vi "Spindle_load_RT_truncated_one(SubVI).vi"() -> (3 "Z_position":string)   [LabVIEW 2017]
uses:
  <vilib>/regexp/Match Regular Expression.xnode
  <vilib>/addons/internet/NI_InternetTK_Core_VIs.lvlib
panel:
  out "speed 3":string
  out "speed 2":string
  out "speed":string
  in  "String 2":string="http://amrcmtconnect.shef.ac.uk:5000/DMU40EVO/current"
  out "content 7":string
  out "after match":string
  out "error out":errorcluster
  out "content 4":string
  out "X_position":string
  out "Y_poistion":string
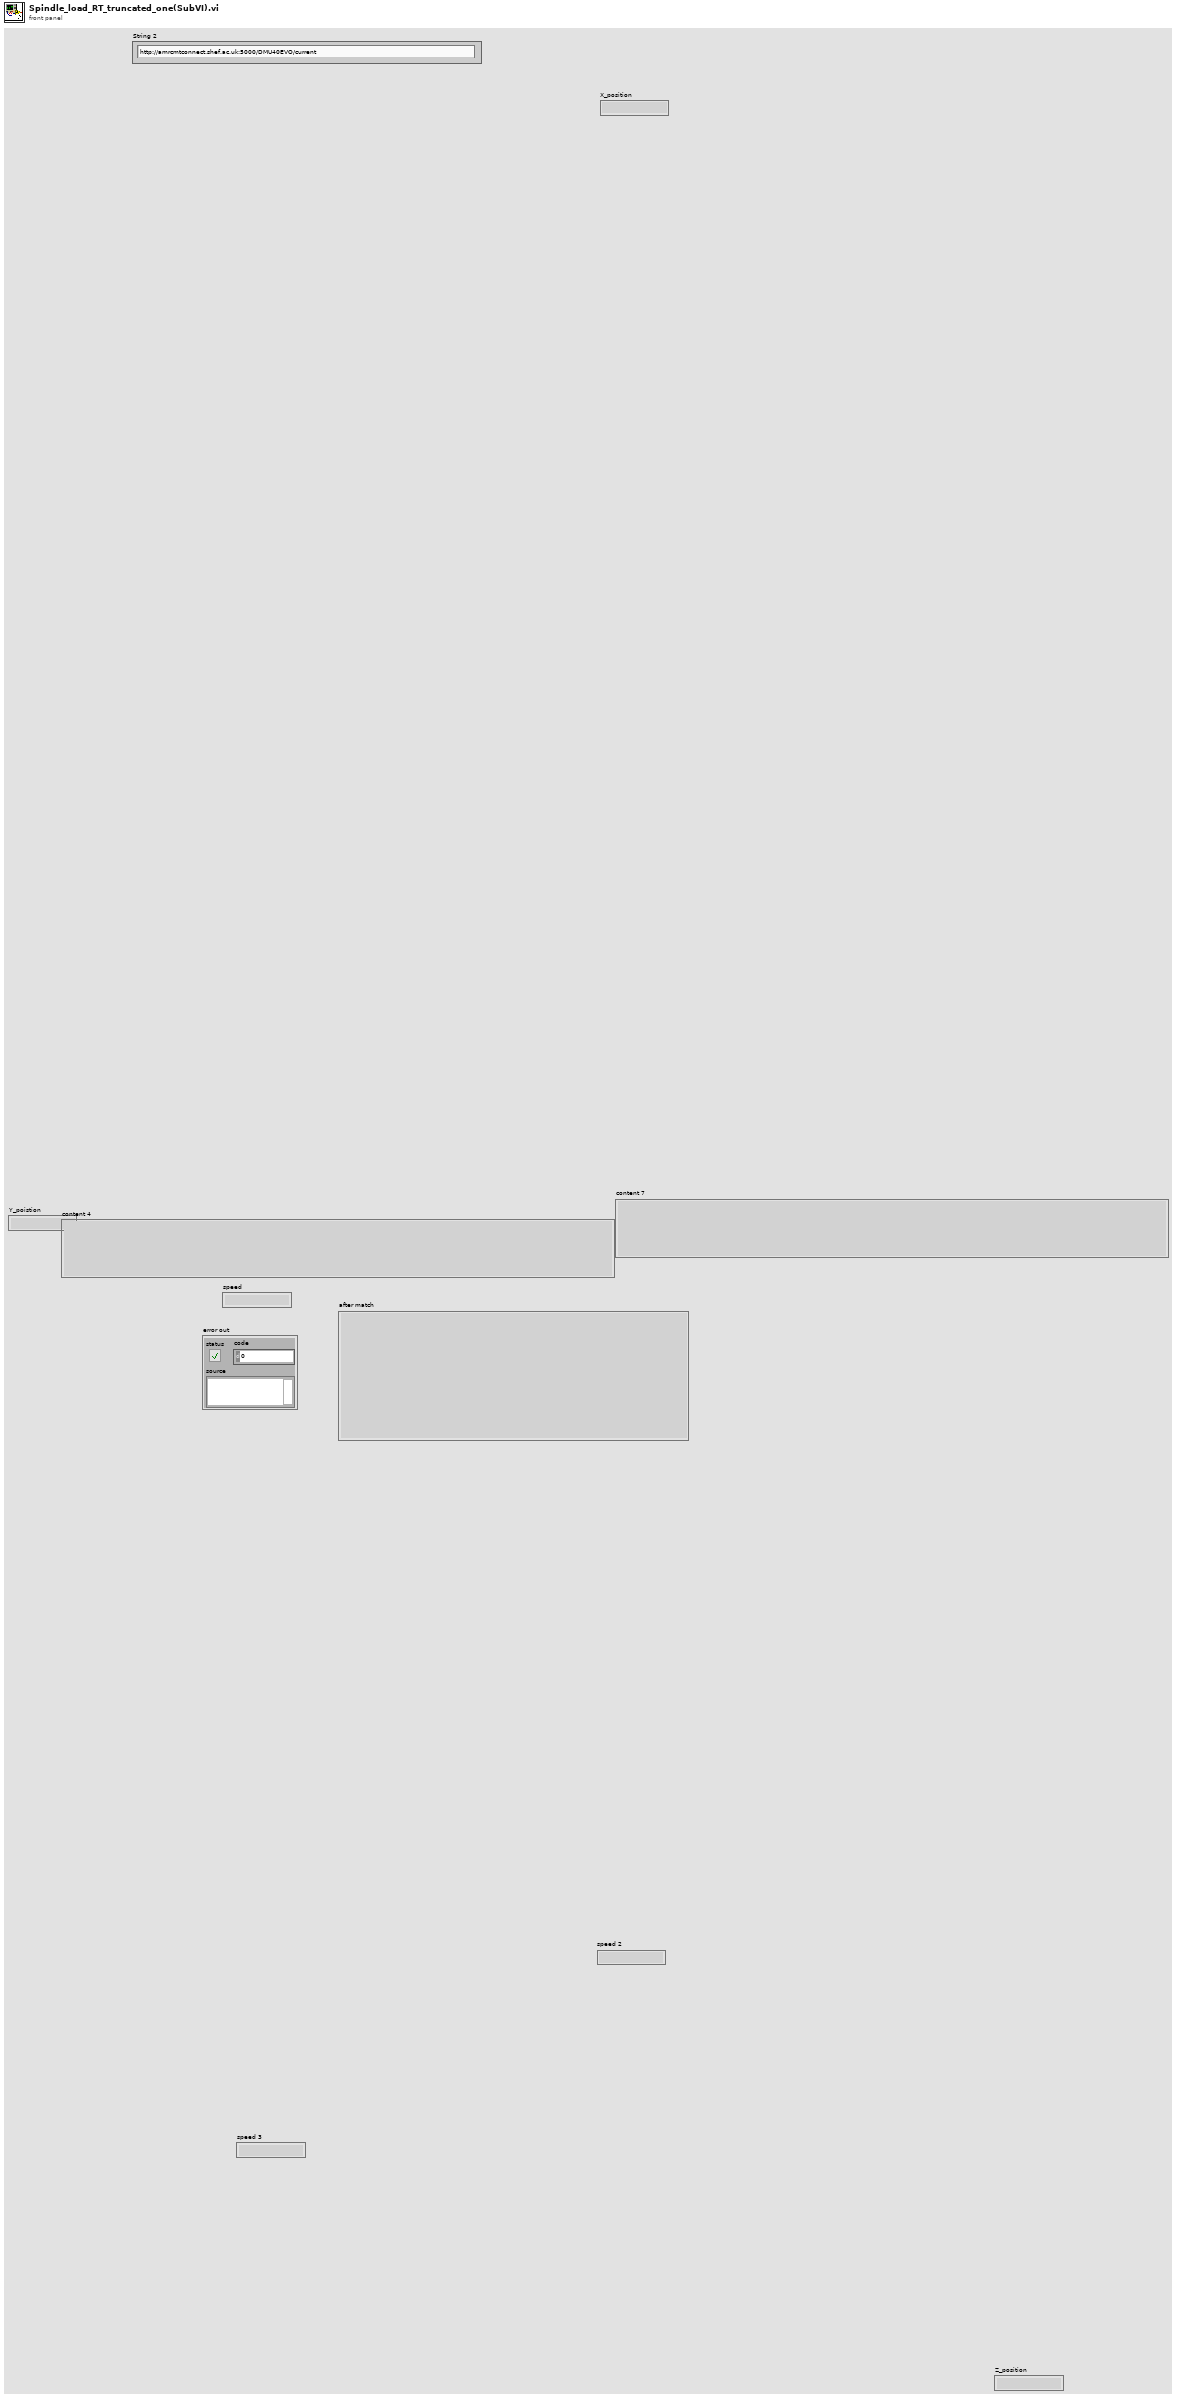
[diagram p1: front panel]
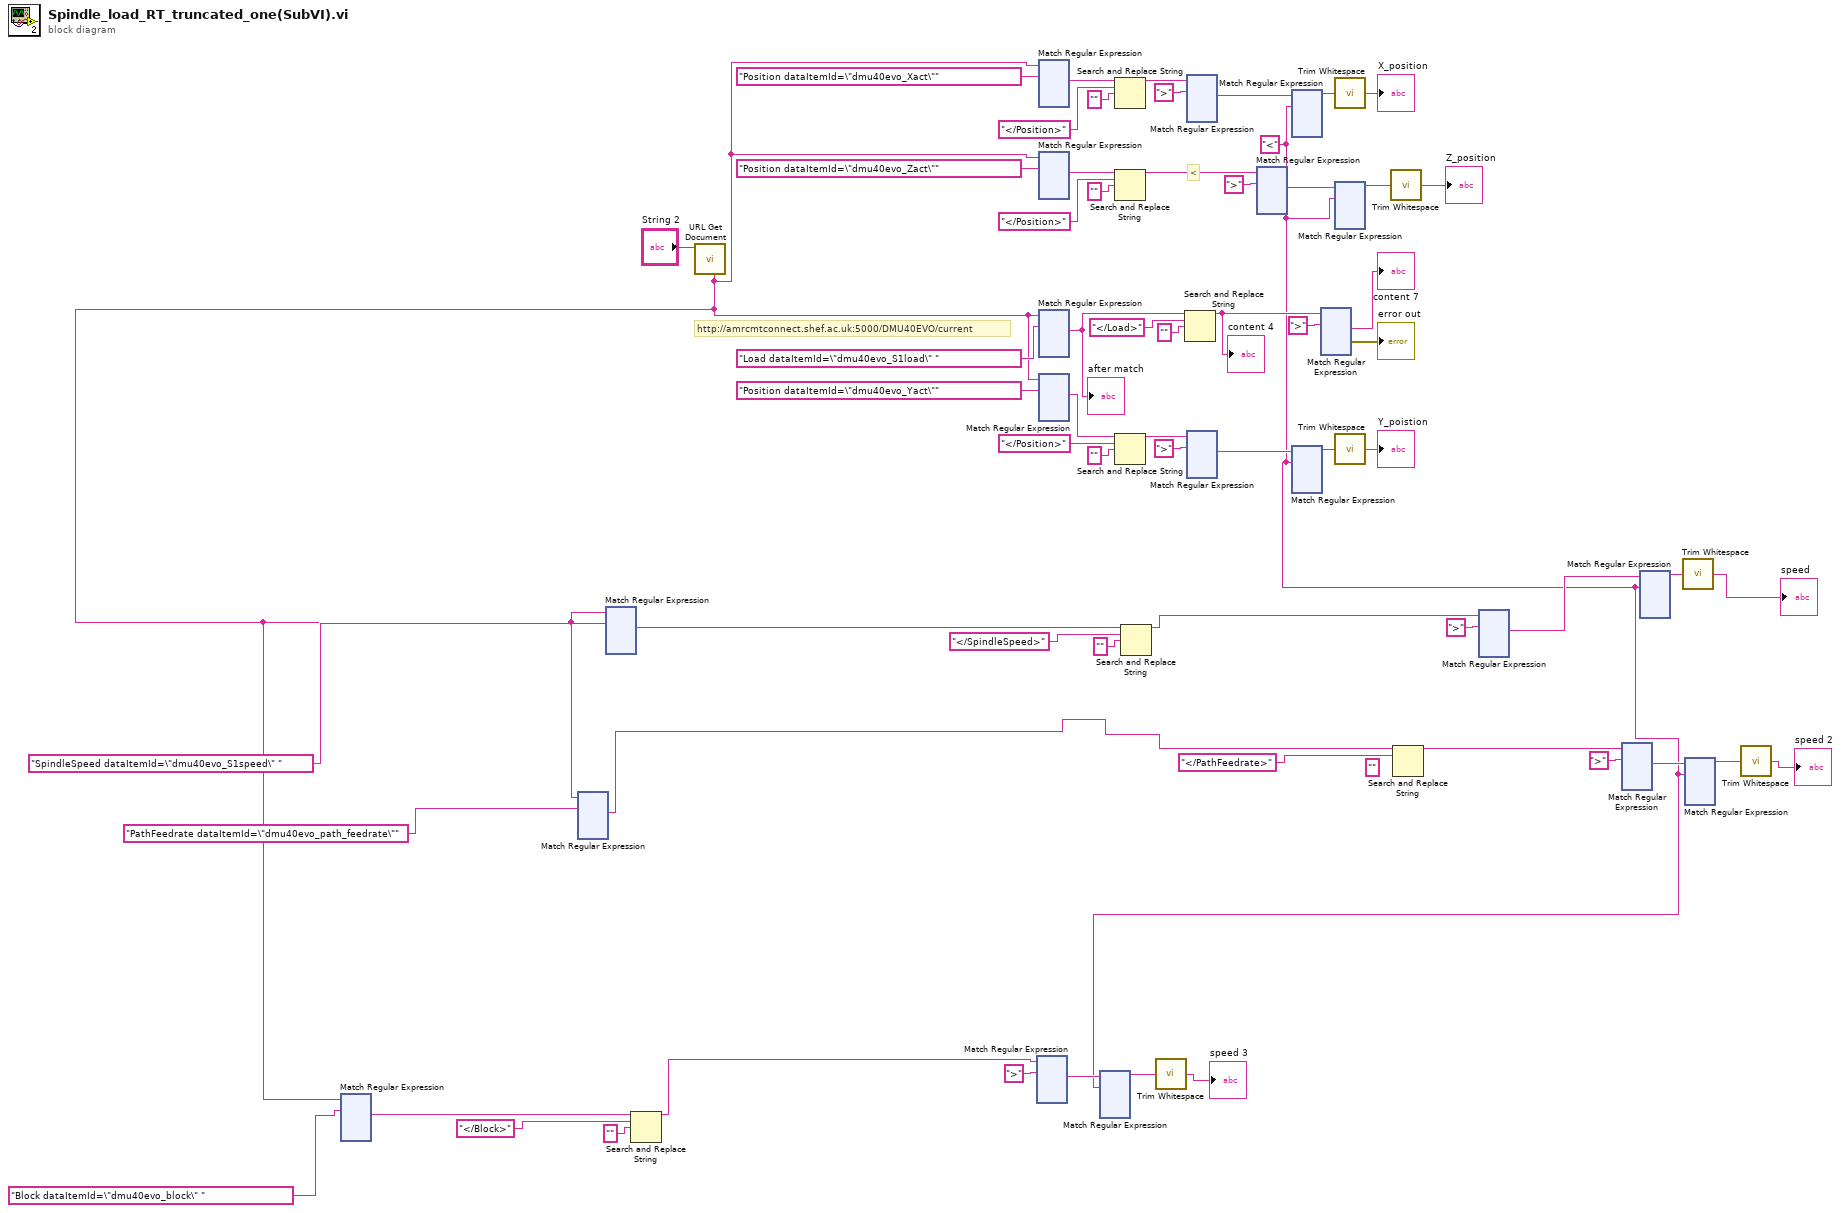
[diagram p0: block diagram]
diagram:
  (unwired) "" ("string")
  w2 = "<" ("string")
  # "http://amrcmtconnect.shef.ac.uk:5000/DMU40EVO/current"
  # "<"
  n1 = call <vilib>:"URL Get Document.vi"("URL"="String 2") -> ("content"=w8:string)  [unwired: 6 in, 4 out]
  n2 = xnode "Match Regular Expression"("input string"=w8, "regular expression"="Block dataItemId=\"dmu40evo_block\" ") -> ("after match"=w7:string)  [unwired: 4 in, 5 out]
  n3 = xnode "Match Regular Expression"("input string"=w8, "regular expression"="PathFeedrate dataItemId=\"dmu40evo_path_feedrate\"") -> ("after match"=w13:string)  [unwired: 4 in, 5 out]
  n4 = xnode "Match Regular Expression"("input string"=w8, "regular expression"="SpindleSpeed dataItemId=\"dmu40evo_S1speed\" ") -> ("after match"=w24:string)  [unwired: 4 in, 5 out]
  n5 = Search and Replace String(input string=w7, search string="</Block>" ("string"), replace string="" ("string")) -> (result string=w1:string)  [unwired: 5 in, 3 out]
  n6 = xnode "Match Regular Expression"("input string"=w1, "regular expression"=">" ("string")) -> ("after match"=w4:string)  [unwired: 4 in, 5 out]
  n7 = xnode "Match Regular Expression"("input string"=w8, "regular expression"="Position dataItemId=\"dmu40evo_Xact\"") -> ("after match"=w38:string)  [unwired: 4 in, 5 out]
  n8 = xnode "Match Regular Expression"("input string"=w8, "regular expression"="Position dataItemId=\"dmu40evo_Zact\"") -> ("after match"=w60:string)  [unwired: 4 in, 5 out]
  n9 = xnode "Match Regular Expression"("input string"=w8, "regular expression"="Load dataItemId=\"dmu40evo_S1load\" ") -> ("after match"=w30:string)  [unwired: 4 in, 5 out]
  "after match" <- w30
  n10 = xnode "Match Regular Expression"("input string"=w8, "regular expression"="Position dataItemId=\"dmu40evo_Yact\"") -> ("after match"=w54:string)  [unwired: 4 in, 5 out]
  n11 = xnode "Match Regular Expression"("input string"=w4, "regular expression"=w2) -> ("before match"=w5:string)  [unwired: 4 in, 5 out]
  n12 = Search and Replace String(input string=w38, search string="</Position>" ("string"), replace string="" ("string")) -> (result string=w41:string)  [unwired: 5 in, 3 out]
  n13 = Search and Replace String(input string=w60, search string="</Position>" ("string"), replace string="" ("string")) -> (result string=w59:string)  [unwired: 5 in, 3 out]
  n14 = Search and Replace String(input string=w54, search string="</Position>" ("string"), replace string="" ("string")) -> (result string=w55:string)  [unwired: 5 in, 3 out]
  n15 = Search and Replace String(input string=w24, search string="</SpindleSpeed>" ("string"), replace string="" ("string")) -> (result string=w23:string)  [unwired: 5 in, 3 out]
  n16 = call <vilib>:"Trim Whitespace.vi"("string"=w5) -> ("trimmed string"=→"speed 3":string)  [unwired: 1 in]
  n17 = Search and Replace String(input string=w30, search string="</Load>" ("string"), replace string="" ("string")) -> (result string=w33:string)  [unwired: 5 in, 3 out]
  "content 4" <- w33
  n18 = xnode "Match Regular Expression"("input string"=w41, "regular expression"=">" ("string")) -> ("after match"=w45:string)  [unwired: 4 in, 5 out]
  n19 = xnode "Match Regular Expression"("input string"=w55, "regular expression"=">" ("string")) -> ("after match"=w48:string)  [unwired: 4 in, 5 out]
  n20 = xnode "Match Regular Expression"("input string"=w59, "regular expression"=">" ("string")) -> ("after match"=w57:string)  [unwired: 4 in, 5 out]
  n21 = xnode "Match Regular Expression"("input string"=w45, "regular expression"=w2) -> ("before match"=w46:string)  [unwired: 4 in, 5 out]
  n22 = xnode "Match Regular Expression"("input string"=w48, "regular expression"=w2) -> ("before match"=w47:string)  [unwired: 4 in, 5 out]
  n23 = xnode "Match Regular Expression"("input string"=w33, "regular expression"=">" ("string")) -> ("after match"=→"content 7":string, "error out"=→"error out":errorcluster)  [unwired: 4 in, 4 out]
  n24 = call <vilib>:"Trim Whitespace.vi"("string"=w46) -> ("trimmed string"=→"X_position":string)  [unwired: 1 in]
  n25 = xnode "Match Regular Expression"("input string"=w57, "regular expression"=w2) -> ("before match"=w56:string)  [unwired: 4 in, 5 out]
  n26 = call <vilib>:"Trim Whitespace.vi"("string"=w47) -> ("trimmed string"=→"Y_poistion":string)  [unwired: 1 in]
  n27 = call <vilib>:"Trim Whitespace.vi"("string"=w56) -> ("trimmed string"=→"Z_position":string)  [unwired: 1 in]
  n28 = Search and Replace String(input string=w13, search string="</PathFeedrate>" ("string")) -> (result string=w20:string)  [unwired: 6 in, 3 out]
  n29 = xnode "Match Regular Expression"("input string"=w23, "regular expression"=">" ("string")) -> ("after match"=w15:string)  [unwired: 4 in, 5 out]
  n30 = xnode "Match Regular Expression"("input string"=w20, "regular expression"=">" ("string")) -> ("after match"=w19:string)  [unwired: 4 in, 5 out]
  n31 = xnode "Match Regular Expression"("input string"=w15, "regular expression"=w2) -> ("before match"=w17:string)  [unwired: 4 in, 5 out]
  n32 = call <vilib>:"Trim Whitespace.vi"("string"=w17) -> ("trimmed string"=→"speed":string)  [unwired: 1 in]
  n33 = xnode "Match Regular Expression"("input string"=w19, "regular expression"=w2) -> ("before match"=w18:string)  [unwired: 4 in, 5 out]
  n34 = call <vilib>:"Trim Whitespace.vi"("string"=w18) -> ("trimmed string"=→"speed 2":string)  [unwired: 1 in]
